vi "UTILITY Read Get Last Dataset.vi"(11 "File Path Control":path) -> (3 "Last Recorded Dataset":string[][](array[string]))   [LabVIEW 2020]
uses:
  <vilib>/Utility/file.llb/Read From Spreadsheet File (string).vi
panel:
  out "Copied Path To Read":path
  out "name":string
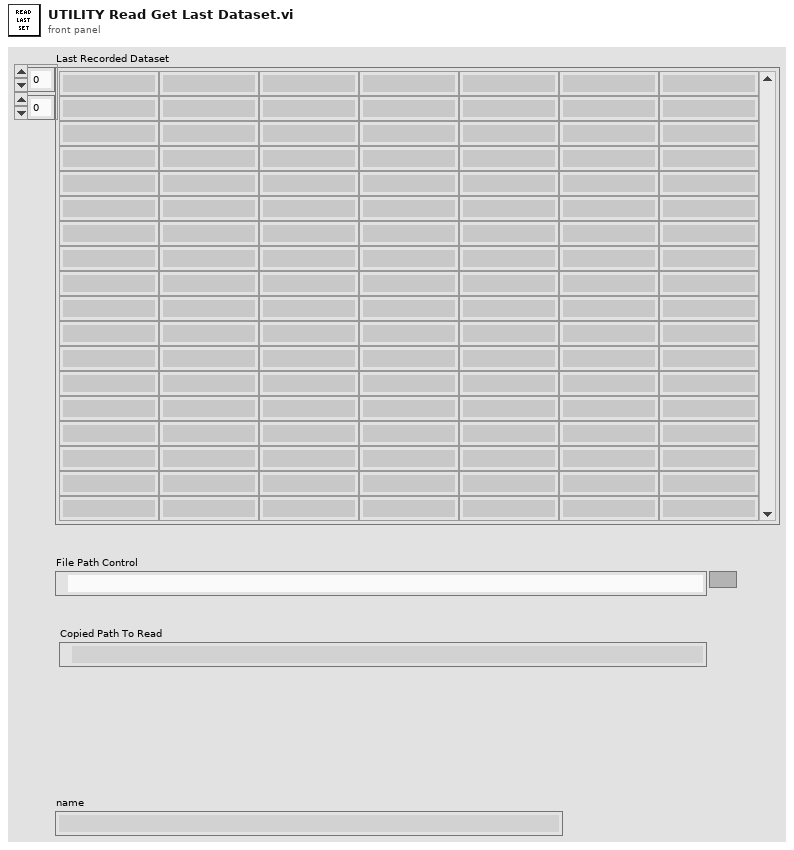
[diagram p1: front panel]
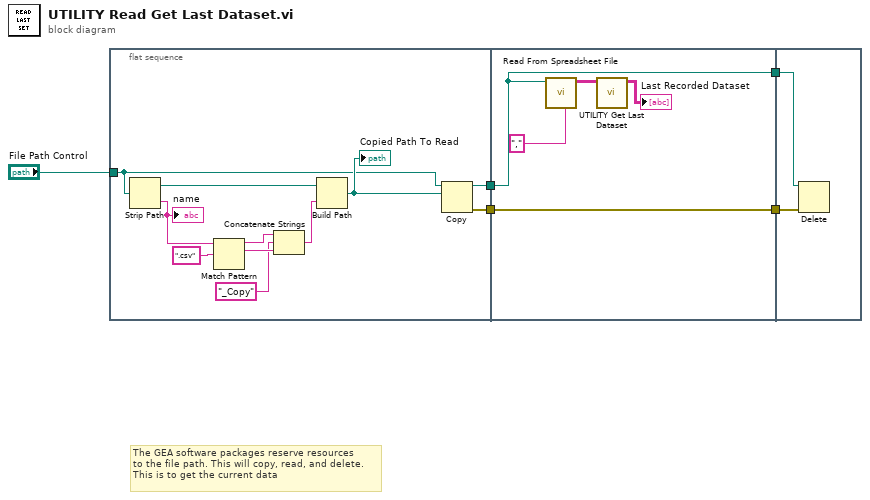
[diagram p0: block diagram]
diagram:
  # "The GEA software packages reserve resources\nto the file path. This will copy, read, and delete.\nThis is to get the current data"
  n1 = flat-sequence {
    tunnel: [w7] -> w5
    tunnel: "File Path Control" -> [w8]
    tunnel: [w6] -> w3
    tunnel: w5 -> [w17]
    tunnel: w3 -> [w18]
    tunnel: [w18] -> w2
    tunnel: [w17] -> w1
    tunnel: w2 -> [w23]
    tunnel: w1 -> [w22]
    frame #0 {
      n2 = Strip Path(path=w8) -> (stripped path=w15:path, name=w9:string)
      "name" <- w9
      n3 = Match Pattern(string=w9, regular expression=".csv") -> (before substring=w11:string, match substring=w13:string)  [unwired: 1 in, 2 out]
      n4 = Concatenate Strings(w11, "_Copy" ("string"), w13) -> (w14:string)
      n5 = Build Path(base path=w15, name or relative path=w14) -> (appended path=w16:path)
      "Copied Path To Read" <- w16
      n6 = Copy(10:w16, 11:w8) -> (0:w6:errorcluster, 3:w7:path)  [unwired: 3 in, 1 out]
    }
    frame #1 {
      n7 = call-poly <vilib>:"Read From Spreadsheet File.vi"("delimiter (\\t)"="," ("delimiter (\\t)"), "file path (dialog if empty)"=w17) -> ("all rows"=w19:string[][])  [unwired: 5 in, 4 out]
      n8 = call "UTILITY Get Last Dataset.vi"("Full Dataset"=w19) -> ("Last Recorded Dataset"=→"Last Recorded Dataset":string[][])  [unwired: 10 in]
    }
    frame #2 {
      n9 = Delete(path (use dialog)=w22, error in=w23) -> ()  [unwired: 3 in, 3 out]
    }
  }
